vi "stop.vi"() -> ()   [LabVIEW 2018]
panel:
  in  "stop":bool
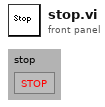
[diagram p1: front panel]
diagram:
